vi "Acc.vi"() -> ()   [LabVIEW 2020]
panel:
  out "data":dynamicdata(graph)
  in  "STOP":bool
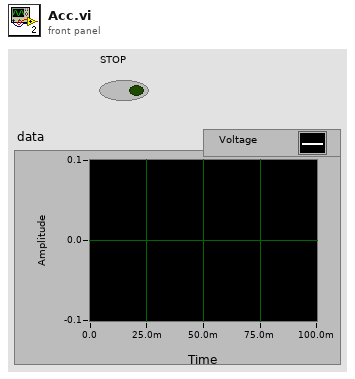
[diagram p1: front panel]
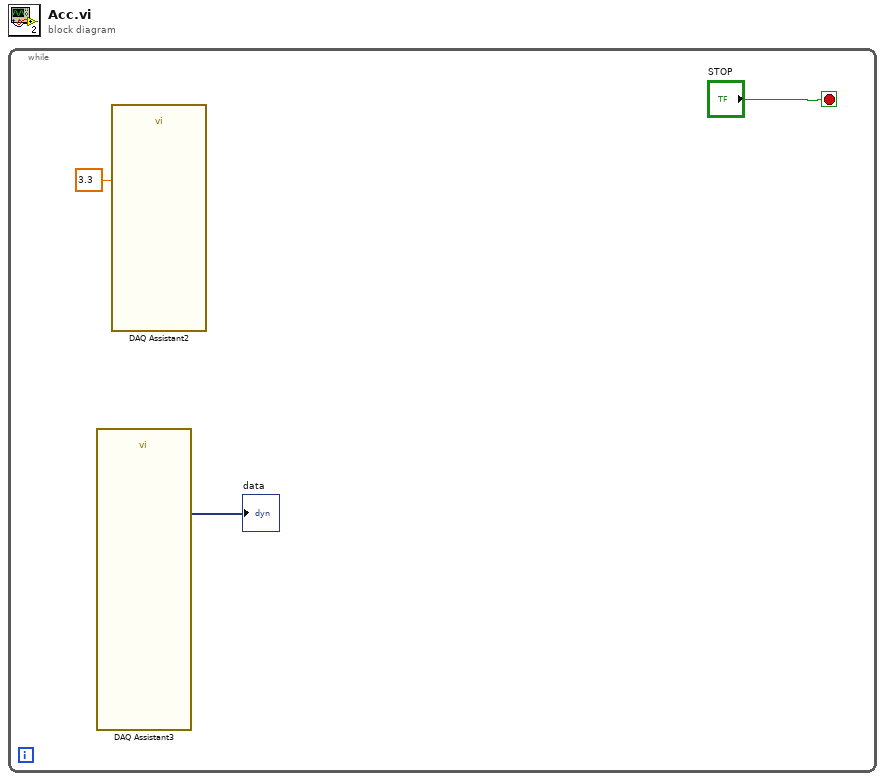
[diagram p0: block diagram]
diagram:
  n1 = while {
    stop <- "STOP" stop-if-true
    n2 = call "DAQ Assistant3"() -> ("data"=→"data":dynamicdata)  [unwired: 16 in, 3 out]
    n3 = call "DAQ Assistant2"("data"=3.3) -> ()  [unwired: 17 in, 2 out]
  }
